vi "Get Restore Point.vi"(7 "Unique ID":string, 8 "error in (no error)":errorcluster, 11 "Test Executive Ref":refnum<data-value>) -> (0 "error out":errorcluster, 1 "Test":refnum<class "Executioner.lvclass">, 3 "Test Executive Ref out":refnum<data-value>, 4 "Restore Point":bool, 5 "Unique ID out":string, 6 "Complete":bool)   [LabVIEW 2019, in "Test Executive.lvlib" / "TestExecutive Ref.lvclass"]
uses:
  <vilib>/gpm_packages/@cs/test-executive/Source/Test Executive/TestExecutive Ref/TestExecutive Ref.lvclass
  <vilib>/gpm_packages/@cs/test-executive/Source/Test Executive/ITestExecutive/ITest Executive.lvclass
  <vilib>/gpm_packages/@cs/test-executive/Source/Test Executive/Executioner/Executioner.lvclass
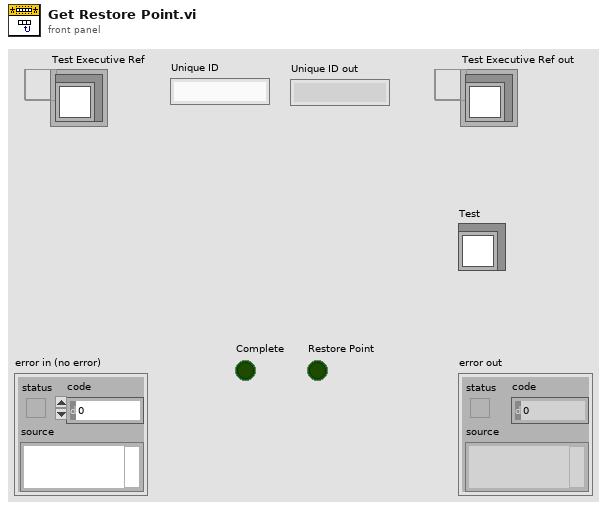
[diagram p1: front panel]
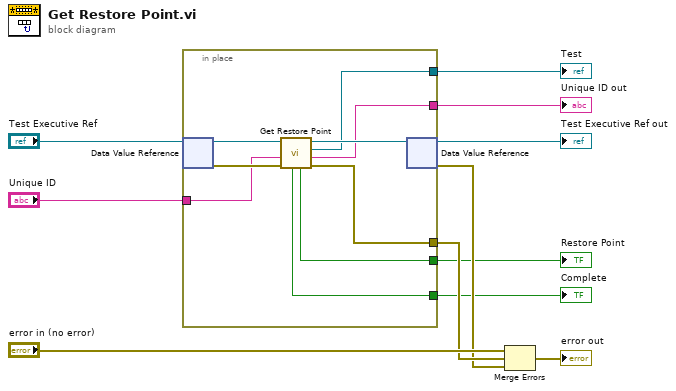
[diagram p0: block diagram]
diagram:
  n1 = in-place {
    in-place-border: "Unique ID" -> [w16]
    in-place-border: [w15] -> w8
    in-place-border: [w19] -> w6
    in-place-border: [w14] -> w3
    in-place-border: [w13] -> w2
    in-place-border: [w12] -> w1
    n2 = in-place-dvr #1("Test Executive Ref") -> (w18:refnum<class "ITest Executive.lvclass">, w20:errorcluster)
    n3 = call-dynamic "Get Restore Point.vi"("error in (no error)"=w20, "Active Unique ID"=w16, "ITest Executive in"=w18) -> ("error out"=w19:errorcluster, "Active Unique ID out"=w15:string, "Test"=w14:refnum<class "Executioner.lvclass">, "ITest Executive out"=w17:refnum<class "ITest Executive.lvclass">, "Restore Point"=w13:bool, "Complete"=w12:bool)  [unwired: 3 in]
    n4 = in-place-dvr #1(w17) -> (→"Test Executive Ref out":refnum<data-value>, w5:errorcluster)
  }
  "Unique ID out" <- w8
  "Test" <- w3
  "Restore Point" <- w2
  "Complete" <- w1
  n5 = Merge Errors("error in (no error)", w6, w5) -> (→"error out":errorcluster)
